vi "RunOperation.vi"(10 "Inputs":string[](array[string]), 11 "Test in":refnum<class "Test.lvclass">) -> (1 "Output/Failure":string, 2 "CLI Process Return Code":i32, 3 "Test out":refnum<class "Test.lvclass">)   [LabVIEW 2014, in "Test.lvclass"]
uses:
  Test.lvclass
  Test.lvclass/Test.ctl
  <vilib>/PNR/Caraya JUnit for Azure Pipelines/JUnit for Azure Pipelines/JUnit for Azure Pipelines.lvclass
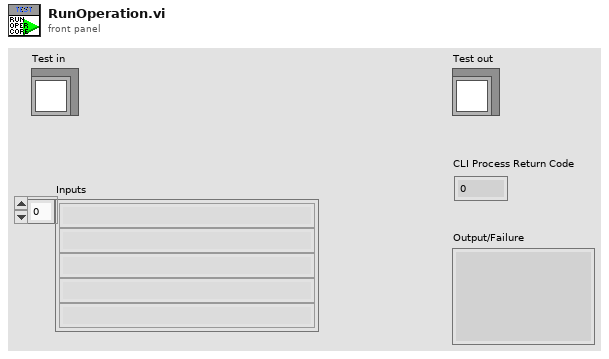
[diagram p1: front panel]
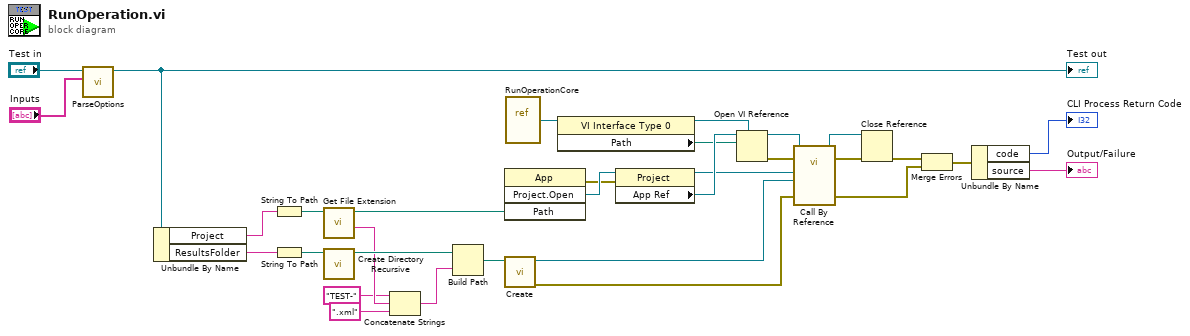
[diagram p0: block diagram]
diagram:
  n1 = call "ParseOptions.vi"("Options"="Inputs", "Test in"="Test in") -> ("Test out"=w28:refnum<class "Test.lvclass">)  [unwired: 8 in, 1 out]
  "Test out" <- w28
  n2 = Unbundle By Name(w28) -> ("Project"=w27:string, "ResultsFolder"=w15:string)
  n3 = String To Path(string=w27) -> (path=w11:path)
  n4 = String To Path(string=w15) -> (path=w13:path)
  n5 = call <vilib>:"Get File Extension.vi"("file"=w11) -> ("filename without extension"=w10:string, "dup file"=w6:path)  [unwired: 7 in, 2 out]
  n6 = call <vilib>:"Create Directory Recursive.vi"("directory"=w13) -> ("directory copy"=w12:path)  [unwired: 4 in, 2 out]
  n7 = Concatenate Strings("TEST-" ("string"), w10, ".xml" ("string")) -> (w7:string)
  n8 = Build Path(base path=w12, name or relative path=w7) -> (appended path=w5:path)
  n9 = invoke class="App" method="Project.Open"("Path"=w6) -> (error out=w16:errorcluster, "Project:Open"=w18:refnum<vi>)  [unwired: 3 in, 2 out]
  n10 = call <vilib>:"Create.vi"("Path"=w5) -> ("error out"=w3:errorcluster, "JUnit for Azure Pipelines"=w4:refnum<class "JUnit for Azure Pipelines.lvclass">)  [unwired: 9 in]
  n11 = vi-ref "RunOperationCore.vi"() -> (w23:refnum<vi>)
  n12 = property class="VI Interface Type 0"(reference=w23) -> (reference out=w21:refnum<vi>, "Path"=w22:path)  [unwired: 1 in, 1 out]
  n13 = property class="Project"(reference=w18, error in=w16) -> (reference out=w17:refnum<vi>, "App Ref"=w24:refnum<vi>)  [unwired: 1 out]
  n14 = Open VI Reference(type specifier VI Refnum (for type only)=w21, application reference (local)=w24, vi path=w22) -> (vi reference=w19:refnum<vi>, error out=w25:errorcluster)  [unwired: 3 in]
  n15 = call-by-ref "?"(reference=w19, error in=w25, 8:"error in (no error)"=w3, "Test Report"=w4, "Project"=w17) -> (reference out=w14:refnum<vi>, error out=w20:errorcluster, 0:"error out"=w1:errorcluster)  [unwired: 8 in]
  n16 = Close Reference(reference=w14, error in (no error)=w20) -> (error out=w26:errorcluster)
  n17 = Merge Errors(w26, w1) -> (w2:errorcluster)
  n18 = Unbundle By Name(w2) -> ("code"=→"CLI Process Return Code":i32, "source"=→"Output/Failure":string)
